vi "Read Label.vi"(8 "error in (no error)":errorcluster, 11 "Panel Object in":refnum<class "Panel Object.lvclass">) -> (0 "error out":errorcluster, 2 "Label":string, 3 "Panel Object out":refnum<class "Panel Object.lvclass">)   [LabVIEW 2018, in "Panel Object.lvclass"]
uses:
  <resource>/dialog/QuickDrop/plugins/PaneRelief/Classes/Panel Object/Panel Object.lvclass
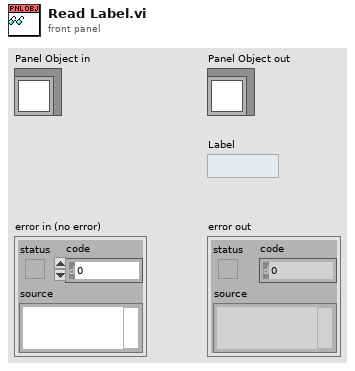
[diagram p1: front panel]
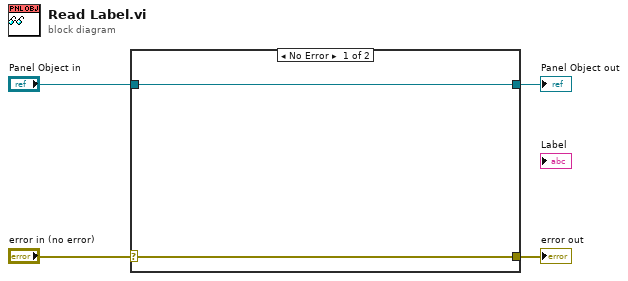
[diagram p0: block diagram]
diagram:
  n1 = case shown="No Error" "error in (no error)" {
    selector: "error in (no error)" -> [w6 w7]
    tunnel: [w6 w7] -> w3
    tunnel: [w5 w8] -> w1
    tunnel: "Panel Object in" -> [w5 w8]
    frame No Error {
    }
    frame Error {
    }
  }
  "error out" <- w3
  "Panel Object out" <- w1
